vi "motorFunction.vi"(0 "VISA Refnum in":refnum<visa-resource-name>, 1 "zone 3 co2":i32, 2 "Light 2":i32, 3 "zone 3 return":i32, 4 "Light 1":i32, 5 "zone 2 co2":i32, 6 "fresh air":i32, 7 "error in (no error)":errorcluster, 8 "Light 3":i32, 9 "zone 1 co2":i32, 10 "zone 2 return":i32, 11 "zone 3 inlet":i32, 12 "zone 2 inlet":i32, 13 "Fans":i32, 14 "zone 1 return":i32, 16 "zone 1 inlet":i32) -> (20 "VISA Refnum out":refnum<visa-resource-name>, 27 "error out":errorcluster)   [LabVIEW 2019]
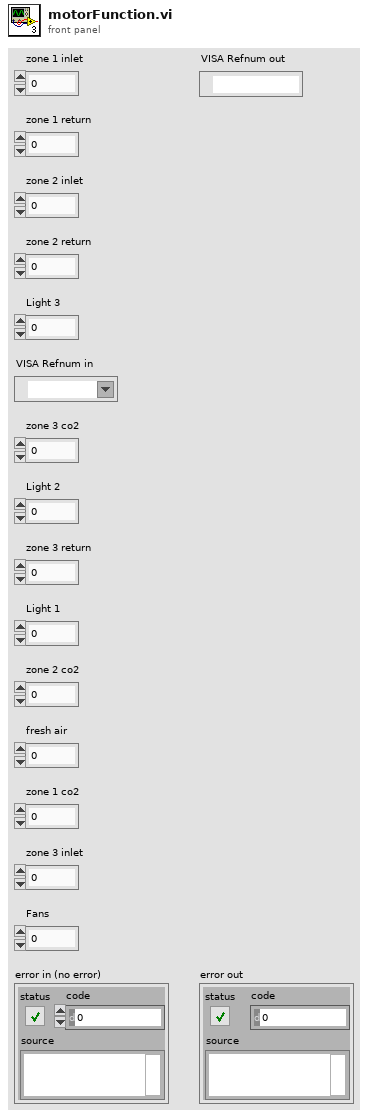
[diagram p1: front panel]
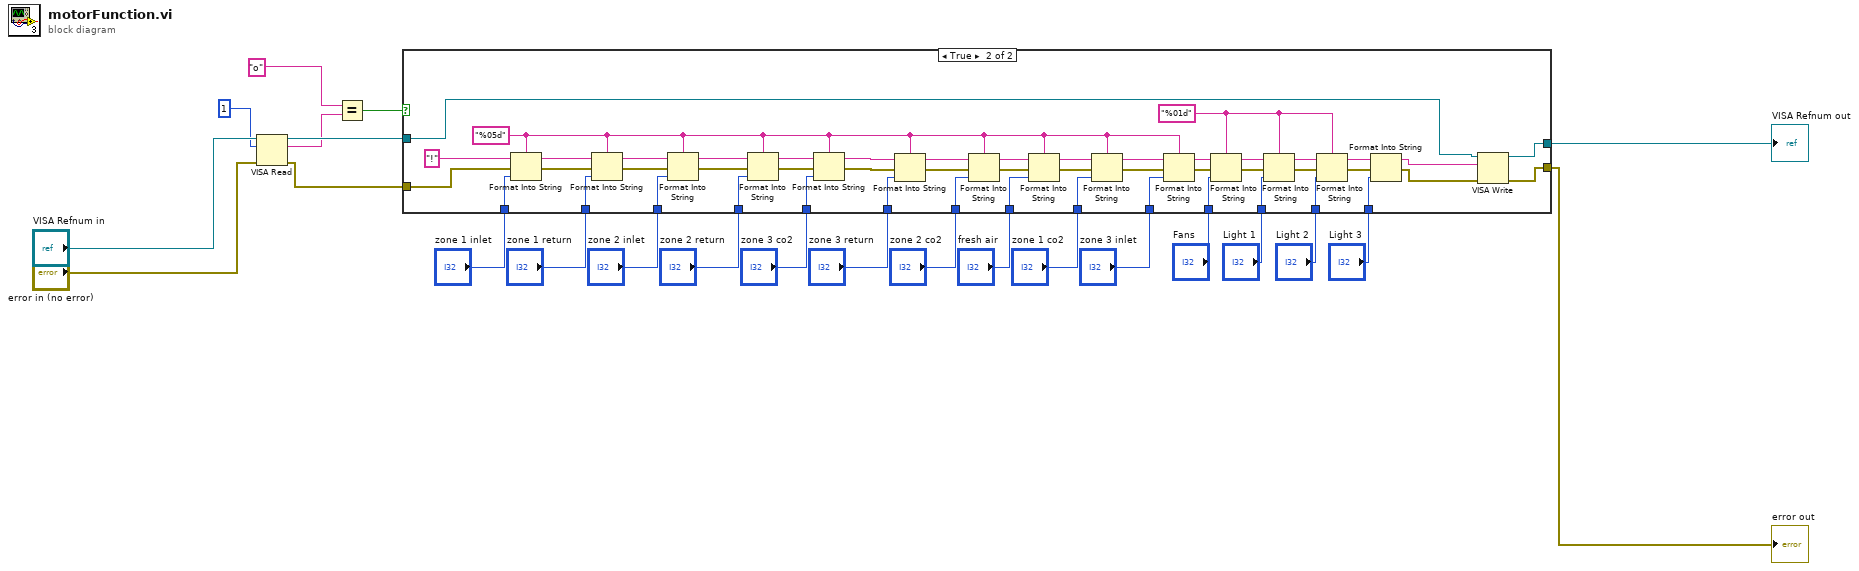
[diagram p0: block diagram]
diagram:
  n1 = VISA Read(VISA resource name="VISA Refnum in", byte count=u32 1, error in (no error)="error in (no error)") -> (VISA resource name out=w24:refnum<visa-resource-name>, read buffer=w4:string, error out=w21:errorcluster)  [unwired: 1 out]
  n2 = Equal?(x="o" ("y"), y=w4) -> (x = y?=w20:bool)
  n3 = case shown="True" w20 {
    tunnel: [w25 w60] -> w23
    tunnel: [w26 w59] -> w22
    tunnel: "zone 1 inlet" -> [_ w42]
    tunnel: "zone 1 return" -> [_ w41]
    tunnel: "zone 2 inlet" -> [_ w40]
    tunnel: "zone 2 return" -> [_ w39]
    tunnel: "zone 3 co2" -> [_ w38]
    tunnel: "zone 3 return" -> [_ w37]
    tunnel: "zone 2 co2" -> [_ w36]
    tunnel: "fresh air" -> [_ w35]
    tunnel: "zone 1 co2" -> [_ w34]
    tunnel: "zone 3 inlet" -> [_ w33]
    tunnel: "Fans" -> [_ w32]
    tunnel: "Light 1" -> [_ w31]
    tunnel: "Light 2" -> [_ w30]
    tunnel: "Light 3" -> [_ w29]
    tunnel: w21 -> [w26 w28]
    tunnel: w24 -> [w25 w27]
    frame False {
    }
    frame True {
      w47 = "%01d" ("format string")
      w54 = "%05d" ("format string")
      n4 = Format Into String(format string=w54, initial string="!" ("write buffer"), error in=w28, w42) -> (resulting string=w74:string, error out=w75:errorcluster)
      n5 = Format Into String(format string=w54, initial string=w74, error in=w75, w41) -> (resulting string=w72:string, error out=w73:errorcluster)
      n6 = Format Into String(format string=w54, initial string=w72, error in=w73, w40) -> (resulting string=w70:string, error out=w71:errorcluster)
      n7 = Format Into String(format string=w54, initial string=w70, error in=w71, w39) -> (resulting string=w68:string, error out=w69:errorcluster)
      n8 = Format Into String(format string=w54, initial string=w68, error in=w69, w38) -> (resulting string=w66:string, error out=w67:errorcluster)
      n9 = Format Into String(format string=w54, initial string=w66, error in=w67, w37) -> (resulting string=w64:string, error out=w65:errorcluster)
      n10 = Format Into String(format string=w54, initial string=w64, error in=w65, w36) -> (resulting string=w63:string, error out=w62:errorcluster)
      n11 = Format Into String(format string=w54, initial string=w63, error in=w62, w35) -> (resulting string=w56:string, error out=w58:errorcluster)
      n12 = Format Into String(format string=w54, initial string=w56, error in=w58, w34) -> (resulting string=w55:string, error out=w57:errorcluster)
      n13 = Format Into String(format string=w54, initial string=w55, error in=w57, w33) -> (resulting string=w50:string, error out=w53:errorcluster)
      n14 = Format Into String(format string=w47, initial string=w50, error in=w53, w32) -> (resulting string=w49:string, error out=w52:errorcluster)
      n15 = Format Into String(format string=w47, initial string=w49, error in=w52, w31) -> (resulting string=w48:string, error out=w51:errorcluster)
      n16 = Format Into String(format string=w47, initial string=w48, error in=w51, w30) -> (resulting string=w45:string, error out=w46:errorcluster)
      n17 = Format Into String(initial string=w45, error in=w46, w29) -> (resulting string=w43:string, error out=w44:errorcluster)  [unwired: 1 in]
      n18 = VISA Write(VISA resource name=w27, write buffer=w43, error in (no error)=w44) -> (VISA resource name out=w60:refnum<visa-resource-name>, error out=w59:errorcluster)  [unwired: 1 out]
    }
  }
  "VISA Refnum out" <- w23
  "error out" <- w22
